vi "FTW-JSON-Format-String.vi"(1 "LabVIEW String":string) -> (0 "JSON String":string)   [LabVIEW 2014]
panel:
  # "Inputs"
  # "Outputs"
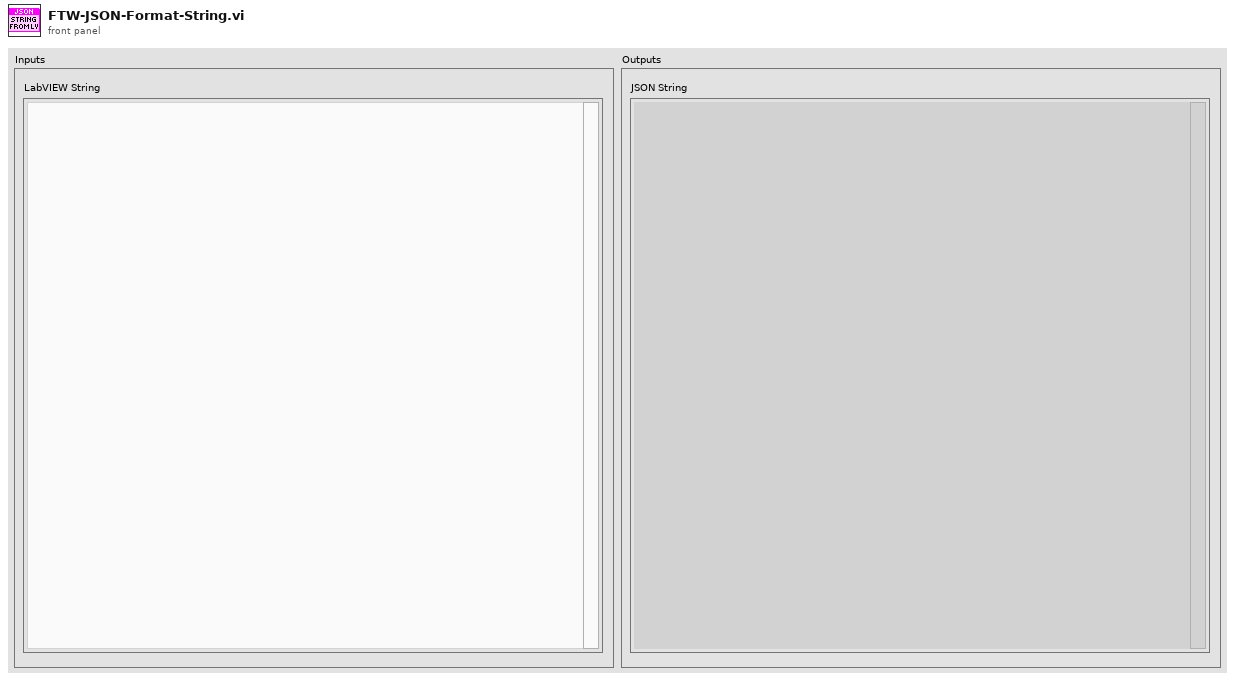
[diagram p1: front panel]
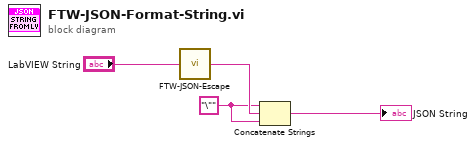
[diagram p0: block diagram]
diagram:
  w1 = "\"" ("string")
  n1 = call "FTW-JSON-Escape.vi"("String"="LabVIEW String") -> ("Escaped UTF-8 String"=w3:string)
  n2 = Concatenate Strings(w1, w3, w1) -> (→"JSON String":string)
